vi "SetControl_EP.vi"(11 "Control":T1) -> (3 "Data":u8[](array[numeric]) format="%x")   [LabVIEW 2014]
uses:
  Control_EP.ctl
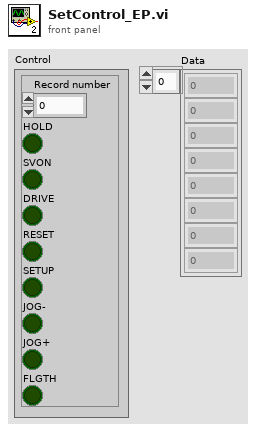
[diagram p1: front panel]
types:
  T1 = typedef "Control_EP.ctl" = cluster{"Record number":u32, "HOLD":bool, "SVON":bool, "DRIVE":bool, "RESET":bool, "SETUP":bool, "JOG-":bool, "JOG+":bool, "FLGTH":bool}
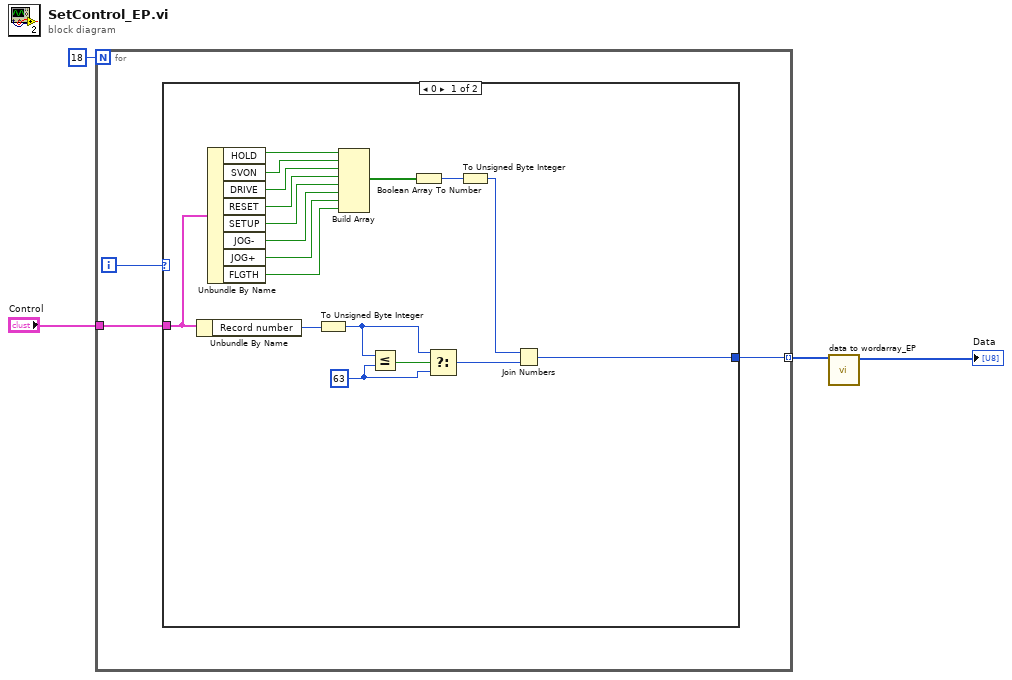
[diagram p0: block diagram]
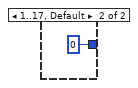
[diagram p2: hidden frame]
diagram:
  n1 = for {
    N: 18 -> [_]
    tunnel: "Control" -> [w6]
    tunnel: [w5] -> w2 mode=indexing
    i -> [w7]
    n2 = case shown="0" w7 {
      tunnel: w6 -> [w10 _]
      tunnel: [w9 u16 0] -> w5
      frame 0 {
        w22 = u8 63 ("y")
        n3 = Unbundle By Name(w10) -> ("Record number"=w25:u32)
        n4 = Unbundle By Name(w10) -> ("HOLD"=w21:bool, "SVON"=w20:bool, "DRIVE"=w19:bool, "RESET"=w18:bool, "SETUP"=w17:bool, "JOG-"=w16:bool, "JOG+"=w15:bool, "FLGTH"=w14:bool)
        n5 = To Unsigned Byte Integer(number=w25) -> (unsigned 8bit integer=w23:u8)
        n6 = Build Array(w21, w20, w19, w18, w17, w16, w15, w14) -> (w13:bool[])
        n7 = Less Or Equal?(x=w23, y=w22) -> (x <= y?=w24:bool)
        n8 = Boolean Array To Number(Boolean array=w13) -> (number=w12:u32)
        n9 = Select(t=w23, s=w24, f=w22) -> (s? t:f=w8:u8)
        n10 = To Unsigned Byte Integer(number=w12) -> (unsigned 8bit integer=w11:u8)
        n11 = Join Numbers(hi=w11, lo=w8) -> ((hi.lo)=w9:u16)
      }
      frame 1..17, Default {
      }
    }
  }
  n12 = call "data to wordarray_EP.vi"("Data"=w2) -> ("Word array"=→"Data":u16[])  [unwired: 10 in]
